vi "Read_OPC_Product_Barcode.vi"(4 "Barcode":u32[](array[numeric])) -> (0 "Counter_Number":i32, 2 "Counter_String":string)   [LabVIEW 2017]
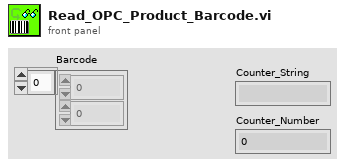
[diagram p1: front panel]
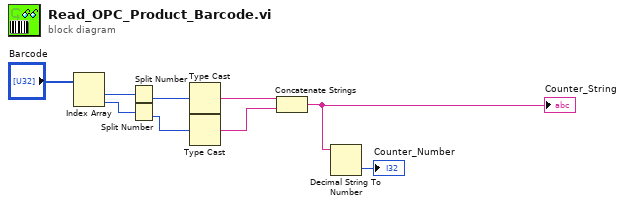
[diagram p0: block diagram]
diagram:
  n1 = Index Array(array="Barcode") -> (element #1=w2:u32, element #2=w1:u32)  [unwired: 2 in]
  n2 = Split Number(x=w2) -> (lo(x)=w4:u16)  [unwired: 1 out]
  n3 = Split Number(x=w1) -> (lo(x)=w3:u16)  [unwired: 1 out]
  n4 = Type Cast(x=w4) -> (*(type *) &x=w7:string)  [unwired: 1 in]
  n5 = Type Cast(x=w3) -> (*(type *) &x=w6:string)  [unwired: 1 in]
  n6 = Concatenate Strings(w7, w6) -> (w5:string)
  "Counter_String" <- w5
  n7 = Decimal String To Number(string=w5) -> (number=→"Counter_Number":i32)  [unwired: 2 in, 1 out]
